vi "交换数组的行(子VI).vi"(11 "输出数组输入":string[][](array[string])) -> (3 "数组":string[](array[string]))   [LabVIEW 2016]
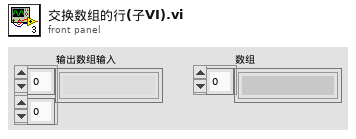
[diagram p1: front panel]
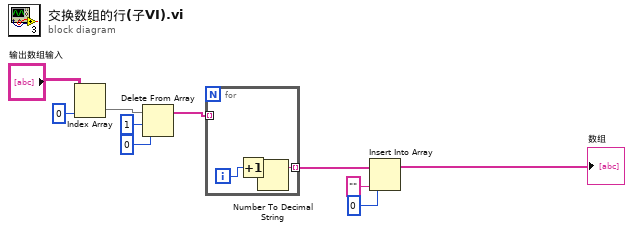
[diagram p0: block diagram]
diagram:
  n1 = Index Array(array="输出数组输入", index (col)=0 ("禁用的索引 (列)")) -> (element=w2:string[])  [unwired: 1 in]
  n2 = Delete From Array(array=w2, length=1 ("长度"), index=0 ("索引")) -> (array with subset deleted=w5:string[])  [unwired: 1 out]
  n3 = for {
    tunnel: w5 -> [_] mode=indexing
    tunnel: [w11] -> w6 mode=indexing
    i -> [w13]
    n4 = Increment(x=w13) -> (x+1=w12:i32)
    n5 = Number To Decimal String(number=w12) -> (decimal integer string=w11:string)  [unwired: 1 in]
  }
  n6 = Insert Into Array(array=w6, index=0 ("索引"), new element="" ("新元素/子数组")) -> (→"数组":string[])
